vi "Main.vi"() -> ()   [LabVIEW 2020]
doc: "This is a home security Vi. Requires Arduino code for some some hardware that is implemented. It alerts the owner when someone enters the password wrong 5 times."
uses:
  Controls/Keyboard.ctl
  Controls/Door Animation.ctl
  Controls/Enum Control.ctl
  <vilib>/userdefined/High Color/IMAQdx.ctl
  <vilib>/MakerHub/LINX/Public/Peripherals/Digital/Digital Write N Chans.vi
  <vilib>/MakerHub/LINX/Private/Local IO/LinxDigitalWrite.vi
  <vilib>/MakerHub/LINX/Public/Utilities/Check Channel.vi
  <vilib>/MakerHub/LINX/Public/Utilities/Open Serial.vi
  <vilib>/MakerHub/LINX/Public/Sensors/Motion/Servo/Servo Open One Channel.vi
  <vilib>/MakerHub/LINX/Private/Utilties/Generate Error.vi
  <vilib>/MakerHub/LINX/Public/Sensors/Motion/Servo/Servo Close One Channel.vi
  <vilib>/MakerHub/LINX/LMH-LINX.lvlib
  <vilib>/vision/driver/NI_Vision_Acquisition_Software.lvlib
  <vilib>/MakerHub/LINX/Public/Sensors/Motion/Servo/Servo.lvlib
panel:
  out "RFID":bool
  in  "Arm/Disarm":bool
  in  "Door Animation":T1
  out "Denied":bool
  out "Granted":bool
  in  "Keyboard":T2
  out "Image":T3(plugin-control)
  in  "QR code":bool
  in  "stop":bool
  out "4x4 pound":string
  out "Passcode Entered":string
  in  "Serial Port":refnum<visa-resource-name>="COM3"
  # "Jaime Alvarez"
  # "ECE 144"
  # "1234 San Diego Bld"
  # "# 7"
  # "Scan your RFID, use QR code,\nor enter password manually\nto unlock the door. \nClap to Arm system or do it\nmanually."
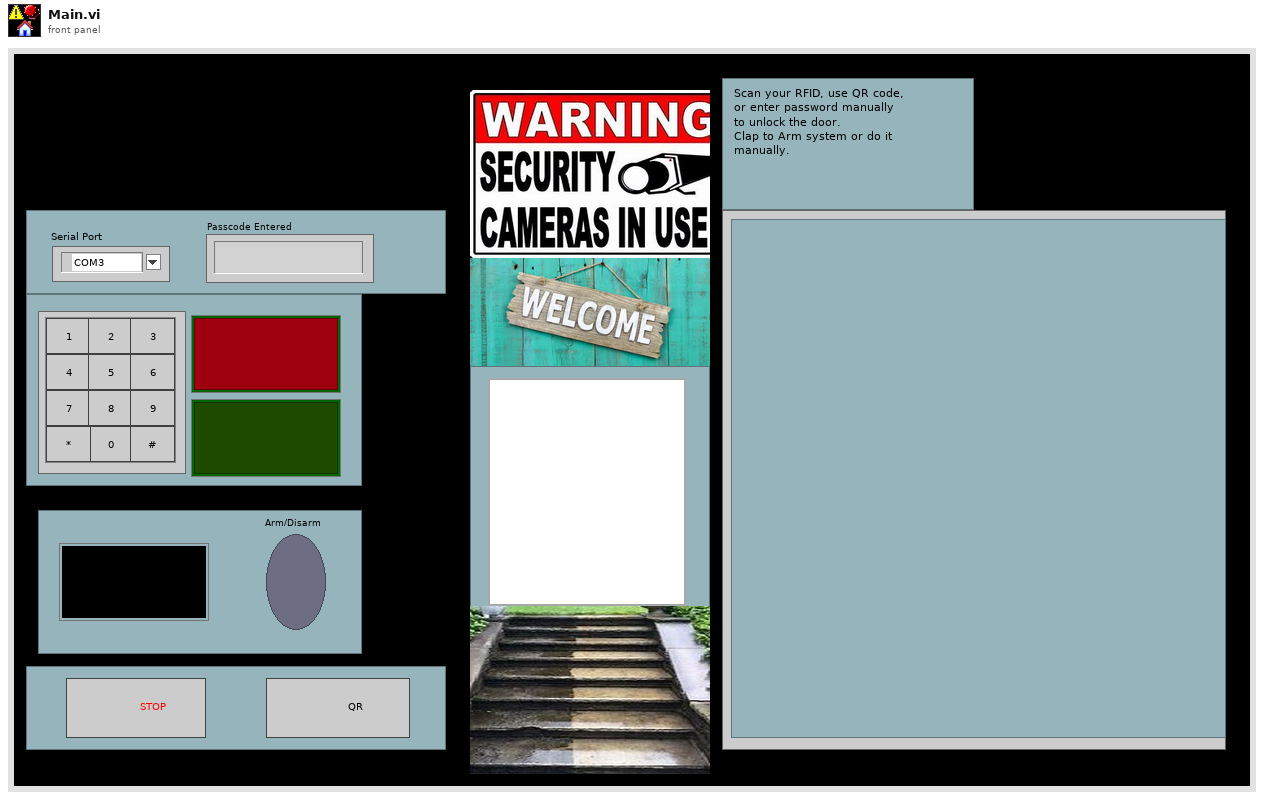
[diagram p1: front panel]
types:
  T1 = typedef "Door Animation.ctl" = u16
  T2 = typedef "Keyboard.ctl" = cluster{"Key 0":bool, "Key 1":bool, "Key 2":bool, "Key 3":bool, "Key 4":bool, "Key 5":bool, "Key 6":bool, "Key 7":bool, "Key 8":bool, "Key 9":bool, "Star Key":bool, "Pound Key":bool}
  T3 = typedef "IMAQ Image.ctl" = refnum<image>
  T4 = cluster{"Correct Song":i32[], "Wrong Song":i32[], "Wrong Beat":i32[]}
  T5 = cluster{"Key0":u8, "key1":u8, "Key2":u8, "Key3":u8, "Key4":u8, "Key5":u8, "Key6":u8, "Key7":u8, "Key8":u8, "Key9":u8, "Key*":u8, "Key#":u8, "Current Key":u8, "Total Code":u8}
  T6 = cluster{"Sound sensor":u8, "RGB":u8[], "Piezo Buzzer":i32, "Servo":i32}
  T7 = typedef "Enum Control.ctl" = enum16{"Initialize", "User Input", "Getting Keys", "Comparing Keys", "Correct Output", "Correct LED", "Wrong LED", "Wrong Output", "Too Many Tries", "Alert Owner", "Turn Off LED", "QR Code", "Stop"}
  T8 = typedef "LMH-LINX.lvlib/LINX Ref.ctl" = cluster{"IO":T9, "Interface":T10, "LINX Device Config":T11}
  T9 = typedef "LMH-LINX.lvlib/Platform.ctl" = enum16{"Remote", "Local"}
  T10 = typedef "LMH-LINX.lvlib/Interface.ctl" = enum16{"Serial", "TCP"}
  T11 = typedef "LMH-LINX.lvlib/Device.lvlib/LINX Device Config.ctl" = cluster{"Interface":T10, "COM Port":refnum<visa-resource-name>, "TCP Configuration":T12, "Device Family":u8, "Device ID":u8, "Device Name":string, "TCP Ref":refnum<k5>, "Channels":T13}
  T12 = typedef "LMH-LINX.lvlib/Device.lvlib/TCP Config.ctl" = cluster{"IP Address":string, "Port":u16}
  T13 = typedef "LMH-LINX.lvlib/Channels.ctl" = cluster{"DI":u8[], "DO":u8[], "AI":u8[], "AO":u8[], "PWM":u8[], "QE":u8[], "UART":u8[], "I2C 2":u8[], "SPI":u8[], "CAN":u8[], "Servo":u8[], "AI Ref (V)":dbl, "AI Resolution (Bits)":u8, "AO Ref (V)":dbl, "AO Resolution (Bits)":u8}
  T14 = enum8{"Enabled", "Disabled", "Disabled and Grayed Out"}
  T15 = typedef "IMAQdx.ctl" = refnum<k21>
  T16 = enum16{"T-Mobile", "AT&T", "Verizon", "Sprint", "Google-Fi"}
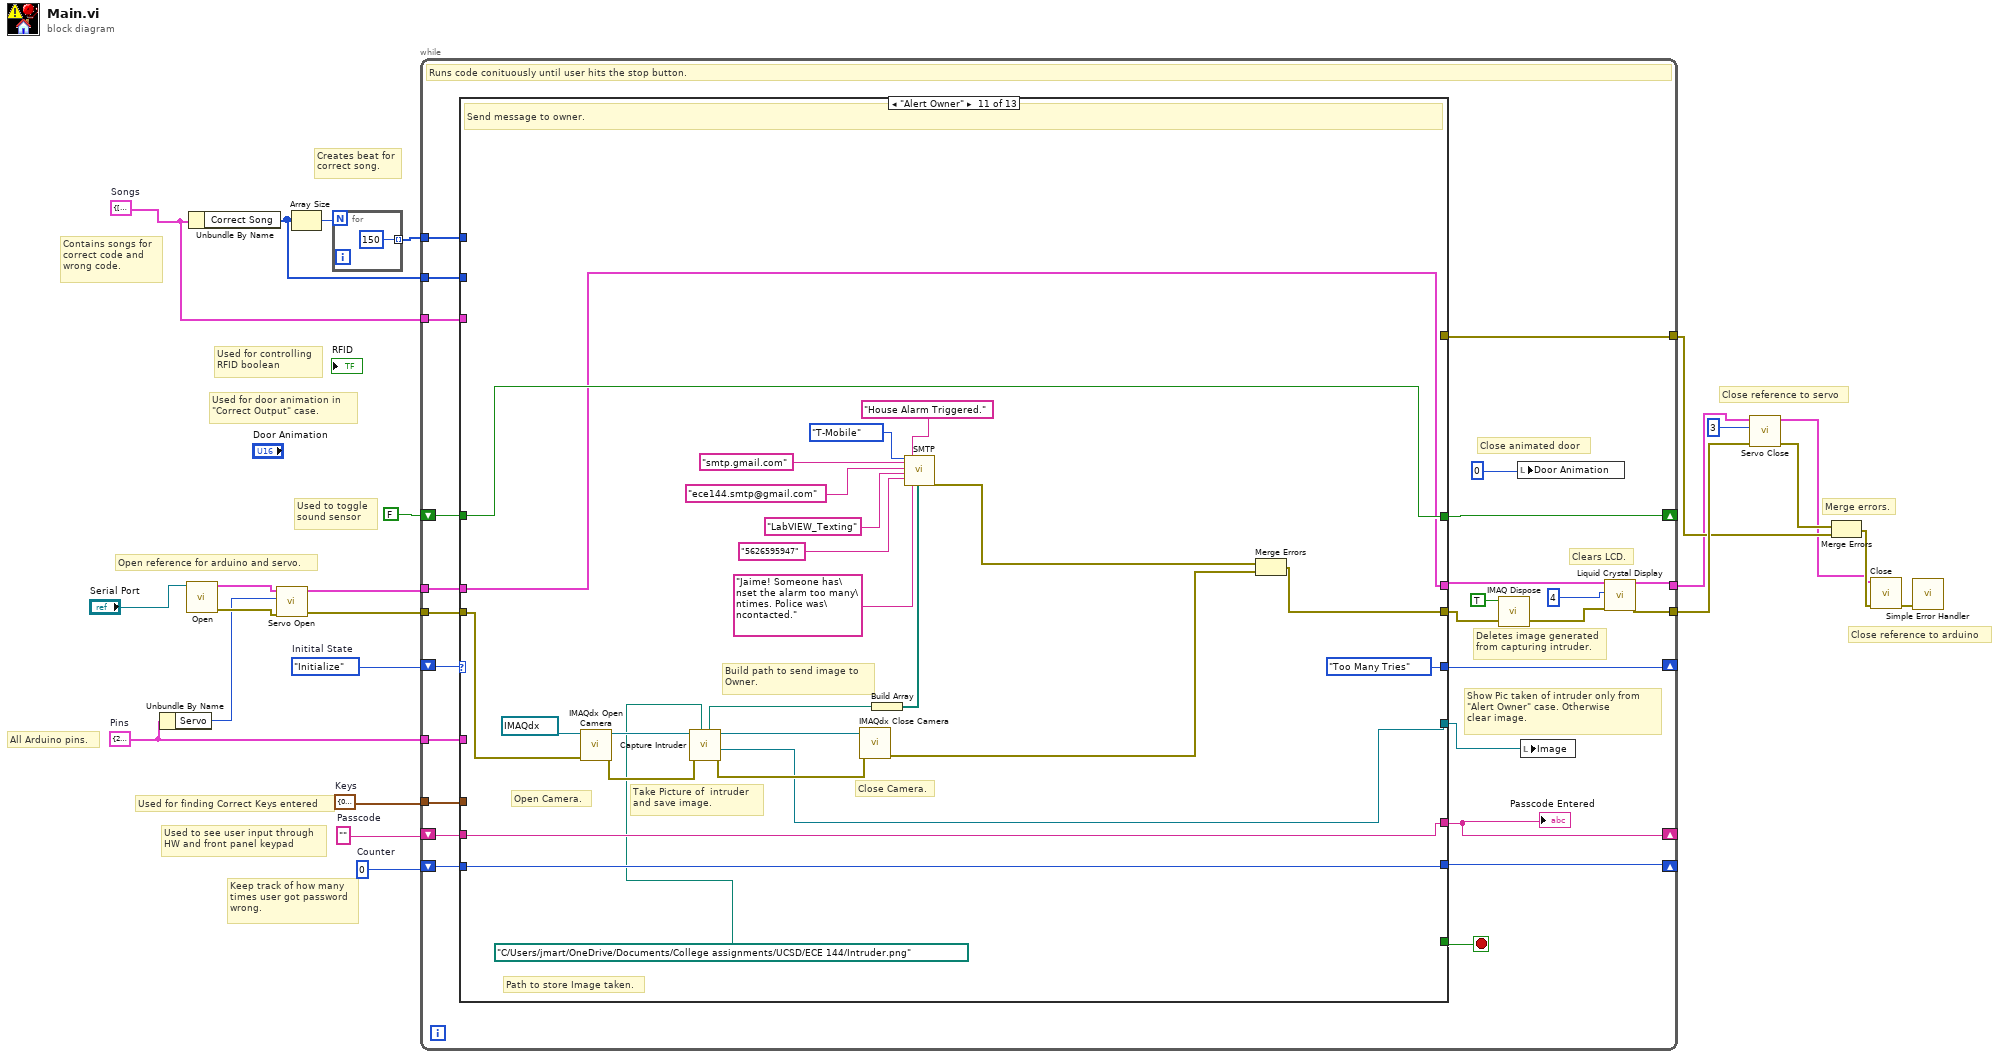
[diagram p0: block diagram]
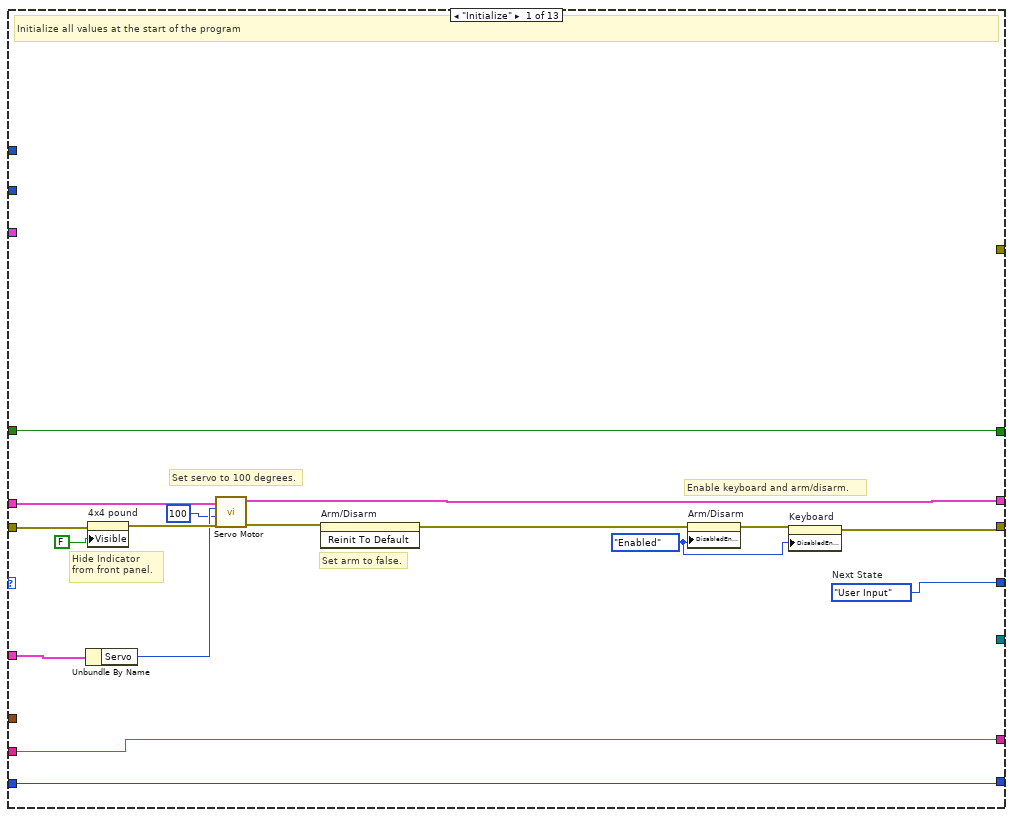
[diagram p2: hidden frame]
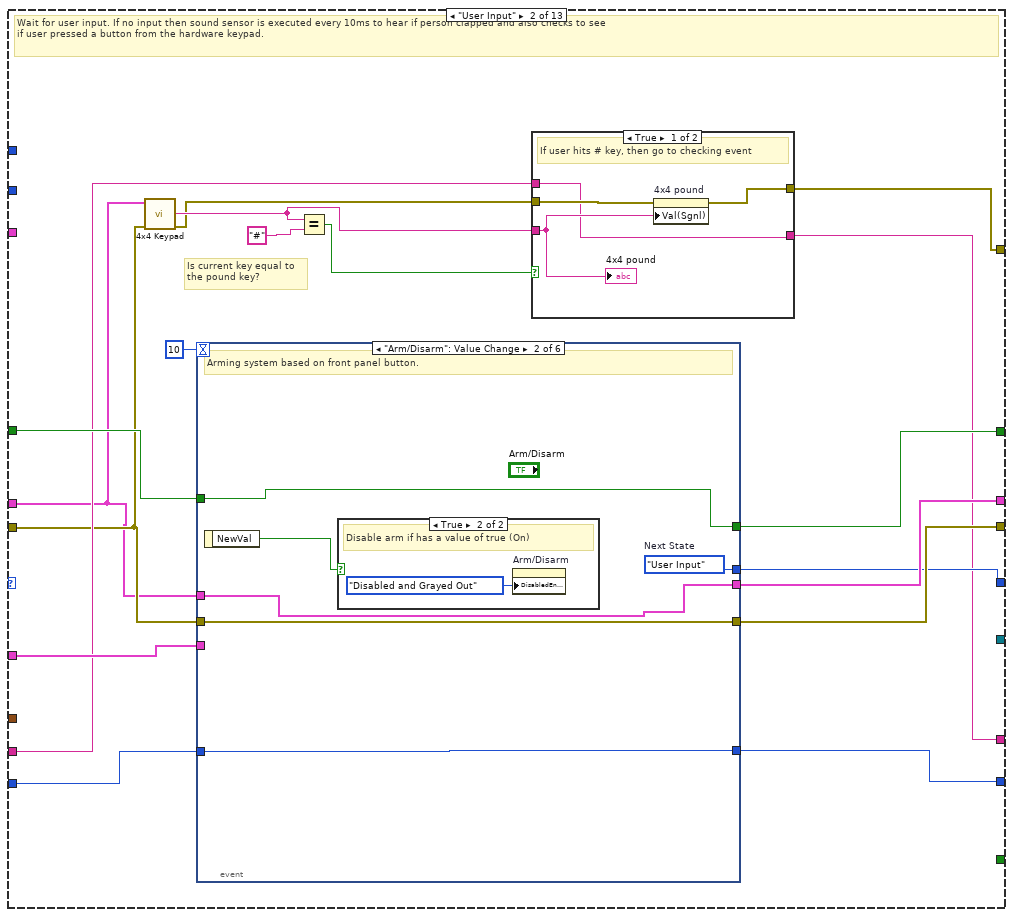
[diagram p3: hidden frame]
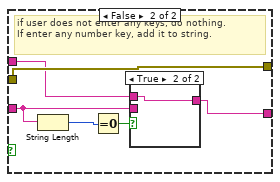
[diagram p4: hidden frame]
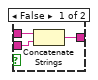
[diagram p5: hidden frame]
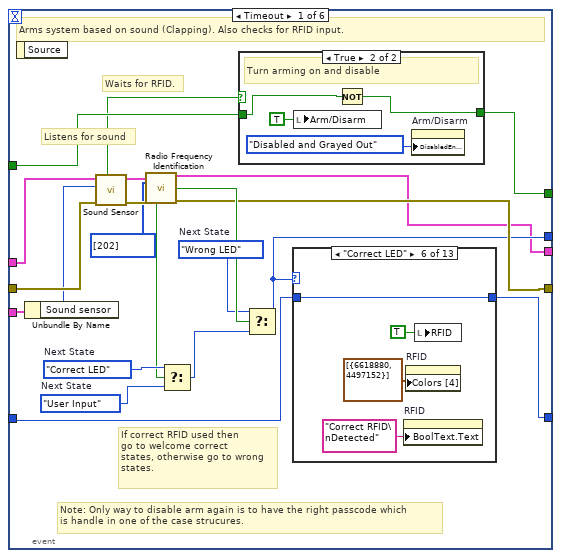
[diagram p6: hidden frame]
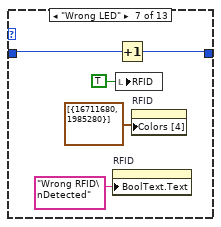
[diagram p12: hidden frame]
diagram:
  w13 = T4 {"Correct Song"=[1319, 1319, 0, 1319, 0, 1047, 1319, 0, 1568, 0, 0, 0, 784, 0, 0, 1568, 0, 0, 659, 0, 0, 880, 0, 988, 0, 932, 0, 880, 784, 1319, 1568, 1760, 0, 1397, 1568, 0, 1319, 0, 1568, 1175, 988, 0, 0], "Wrong Song"=[262, 523, 220, 440, 233, 466, 0, 0, 262, 523, 220, 440, 233, 466, 0, 0, 175, 349, 147, 294, 156, 311, 0, 0, 311, 277, 294, 277, 311, 311, 208, 208, 277, 262, 370, 349, 165, 466, 440, 415, 311, 247, 233, 220, 208, 0, 0, 0], "Wrong Beat"=[250, 250, 250, 250, 250, 250, 500, 1000, 250, 250, 250, 250, 250, 250, 500, 1000, 250, 250, 250, 250, 250, 250, 500, 1000, 250, 250, 250, 250, 250, 250, 500, 500, 250, 250, 250, 500, 500, 500, 500, 250, 250, 250, 250, 250, 250, 500, 500, 500]}  # Songs
  w19 = 0  # Counter
  w20 = ""  # Passcode
  w21 = T5 {"Key0"=0, "key1"=1, "Key2"=2, "Key3"=3, "Key4"=4, "Key5"=5, "Key6"=6, "Key7"=7, "Key8"=8, "Key9"=9, "Key*"=10, "Key#"=11, "Current Key"=0, "Total Code"=0}  # Keys
  w8 = T6 {"Sound sensor"=2, "RGB"=[45, 46, 47], "Piezo Buzzer"=9, "Servo"=3}  # Pins
  w23 = Enum_Control."Initialize"  # Initital State
  # "Used for controlling\nRFID boolean"
  # "Merge errors."
  # "Close reference to servo"
  # "Close reference to arduino"
  # "Contains songs for\ncorrect code and\nwrong code."
  # "Used for door animation in \n\"Correct Output\" case."
  # "Open reference for arduino and servo."
  # "Creates beat for\ncorrect song."
  # "Used to toggle \nsound sensor"
  # "Used to see user input through\nHW and front panel keypad"
  # "All Arduino pins."
  # "Used for finding Correct Keys entered"
  # "Keep track of how many\ntimes user got password\nwrong."
  n1 = Unbundle By Name(w8) -> ("Servo"=w7:i32)
  n2 = call-poly <vilib>:"Open.vi"("Serial Port"="Serial Port") -> ("Error Out"=w9:errorcluster, "LINX Resource"=w10:T8)  [unwired: 8 in, 1 out]
  n3 = Unbundle By Name(w13) -> ("Correct Song"=w14:i32[])
  n4 = call-poly <vilib>:"Servo Open.vi"("Error In"=w9, "Servo Channel"=w7, "LINX Resource"=w10) -> ("Error Out"=w11:errorcluster, "LINX Resource"=w12:T8)  [unwired: 7 in]
  n5 = Array Size(array=w14) -> (size(s)=w16:i32)
  n6 = for {
    N: w16 -> [_]
    tunnel: [150] -> w15 mode=indexing
  }
  n7 = while {
    shift-right: [w50] -> _
    shift-left: w23 -> [w51]
    tunnel: w12 -> [w49]
    tunnel: w11 -> [w48]
    shift-right: [w46] -> _
    shift-left: FALSE -> [w47]
    tunnel: [w39] -> w5
    tunnel: [w37] -> w2
    tunnel: w8 -> [w45]
    tunnel: w21 -> [w44]
    shift-right: [w42] -> _
    shift-left: w20 -> [w43]
    shift-right: [w40] -> _
    shift-left: w19 -> [w41]
    tunnel: [w35] -> w4
    tunnel: w15 -> [w33]
    tunnel: w14 -> [w32]
    tunnel: w13 -> [w31]
    stop <- w34 stop-if-true
    # "Deletes image generated\nfrom capturing intruder."
    # "Close animated door"
    # "Show Pic taken of intruder only from\n\"Alert Owner\" case. Otherwise\nclear image."
    # "Clears LCD."
    # "Runs code conituously until user hits the stop button."
    n8 = case shown="\"Alert Owner\"" w51 {
      tunnel: [w68 w82 w184 w200 w236 w252 w261 w304 w361 w403 Enum_Control."Too Many Tries" ("Initital State") Enum_Control."User Input" ("Initital State") w481] -> w50
      tunnel: w49 -> [w58 w70 w191 w199 w247 w257 w275 w299 w359 w401 w441 w476 w483]
      tunnel: w48 -> [w60 w71 w190 w215 w245 _ w272 w298 w356 w373 w436 w474 w482]
      tunnel: w47 -> [w67 w85 w192 w206 w248 w251 w268 w292 w362 w374 w454 w471 w484]
      tunnel: [w67 w80 w192 w206 w248 w251 w268 w292 w362 w374 w454 w471 w484] -> w46
      tunnel: [w61 w83 w185 w214 w244 w249 w266 w279 w344 w366 w444 w462 w482] -> w27
      tunnel: [w57 w84 w191 w199 w247 w253 w270 w276 w343 w387 w441 w475 w483] -> w36
      tunnel: [_ _ _ _ _ _ _ _ _ _ _ _ TRUE] -> w34
      tunnel: w45 -> [w54 w81 _ _ _ w256 w274 w284 _ w380 _ w478 _]
      tunnel: w44 -> [_ _ w189 _ _ _ _ _ _ _ _ _ _]
      tunnel: w43 -> [w65 w73 w188 w207 w235 w255 w269 w303 w360 w402 w452 w466 _]
      tunnel: [w65 w72 w178 w207 w243 w255 w269 w303 w360 w402 w452 w466 "" ("Passcode")] -> w42
      tunnel: w41 -> [w64 w79 w183 w208 w240 w254 w260 _ w341 _ w451 w470 _]
      tunnel: [w64 w78 w183 w208 w240 w254 w260 0 ("Counter") w341 0 ("Counter") w451 w470 0 ("Counter")] -> w40
      tunnel: [_ w69 _ _ _ _ _ w280 _ w375 _ _ _] -> w35
      tunnel: w33 -> [_ _ _ _ _ _ _ w291 _ _ _ _ _]
      tunnel: w32 -> [_ _ _ _ _ _ _ w290 _ _ _ _ _]
      tunnel: w31 -> [_ _ _ _ _ _ _ _ _ w381 _ _ _]
      tunnel: [_ _ _ _ _ _ _ _ _ _ w442 _ _] -> w29
      frame "Initialize" {
        w62 = T14."Enabled" ("Disabled")
        w68 = Enum_Control."User Input"  # Next State
        # "Set servo to 100 degrees."
        # "Set arm to false."
        # "Enable keyboard and arm/disarm."
        # "Hide Indicator\nfrom front panel."
        # "Initialize all values at the start of the program"
        n9 = Unbundle By Name(w54) -> ("Servo"=w53:i32)
        n10 = property on="4x4 pound" class="Str"(error in=w60, "Visible"=FALSE) -> (error out=w56:errorcluster)  [unwired: 1 in, 1 out]
        n11 = call "Servo Motor.vi"("Error In"=w56, "Position"=100, "Servo Channel"=w53, "LINX Resource In"=w58) -> ("Error Out"=w55:errorcluster, "LINX Resource Out"=w57:T8)  [unwired: 5 in, 1 out]
        n12 = invoke on="Arm/Disarm" class="Bool (strict)" method="Reinit To Default"(error in=w55) -> (error out=w66:errorcluster)  [unwired: 2 in, 2 out]
        n13 = property on="Arm/Disarm" class="Bool (strict)"(error in=w66, "DisabledEnum"=w62) -> (error out=w63:errorcluster)  [unwired: 1 in, 1 out]
        n14 = property on="Keyboard" class="Clust (strict)"(error in=w63, "DisabledEnum"=w62) -> (error out=w61:errorcluster)  [unwired: 1 in, 1 out]
      }
      frame "User Input" {
        # "Is current key equal to \nthe pound key?"
        # "Wait for user input. If no input then sound sensor is executed every 10ms to hear if person clapped and also checks to see\nif user pressed a button from the hardware keypad."
        n15 = call "4x4 Keypad.vi"("Error In"=w71, "LINX Resource"=w70) -> ("Error Out"=w74:errorcluster, "string out"=w75:string)  [unwired: 7 in, 1 out]
        n16 = event shown="[1] \"Arm/Disarm\": Value Change" {
          selector: _ -> [_ _ _ _ _ _]
          dyn-events: _ -> [_ _ _ _ _ _]
          timeout: 10 -> [_ _ _ _ _ _]
          tunnel: [w104 w152 w159 w166 w169 w177] -> w82
          tunnel: w85 -> [w119 w147 w154 w162 w172 w176]
          tunnel: w70 -> [w121 w148 w156 w161 w171 w175]
          tunnel: w71 -> [w120 w149 w155 w160 w170 w174]
          tunnel: [w118 w147 w154 w162 w172 w176] -> w80
          tunnel: [w101 w148 w156 w161 w171 w175] -> w84
          tunnel: [w106 w149 w155 w160 w170 w174] -> w83
          tunnel: w81 -> [w117 _ _ _ _ _]
          tunnel: w79 -> [w105 w150 w157 w164 w168 w173]
          tunnel: [w103 w150 w157 w163 w167 w173] -> w78
          event Timeout {
            w108 = Enum_Control."Wrong LED"  # Next State
            w112 = Enum_Control."Correct LED"  # Next State
            w111 = Enum_Control."User Input"  # Next State
            # "Waits for RFID."
            # "Listens for sound"
            # "If correct RFID used then \ngo to welcome correct\nstates, otherwise go to wrong\nstates."
            # "Note: Only way to disable arm again is to have the right passcode which\nis handle in one of the case strucures."
            # "Arms system based on sound (Clapping). Also checks for RFID input."
            n17 = event-data() -> ()  [unwired: 1 in, 1 out]
            n18 = Unbundle By Name(w117) -> ("Sound sensor"=w116:u8)
            n19 = call "Sound Sensor.vi"("Error In"=w120, "DI Channel"=w116, "LINX Resource In"=w121) -> ("Error Out"=w114:errorcluster, "Sound?"=w113:bool, "LINX Resource Out"=w115:T8)  [unwired: 6 in]
            n20 = call "Radio Frequency Identification.vi"("LINX Resource"=w115, "RFID Value"=u8[] [202], "Error In"=w114) -> ("LINX Resource Out"=w101:T8, "Wrong ID"=w109:bool, "Correct ID"=w107:bool, "Error Out"=w106:errorcluster)  [unwired: 8 in, 1 out]
            n21 = Select(t=w112, s=w107, f=w111) -> (s? t:f=w110:T7)
            n22 = case shown="True" w113 {
              tunnel: w119 -> [w142 w145]
              tunnel: [w142 w146] -> w118
              frame False {
                # "Do nothing."
              }
              frame True {
                # "Turn arming on and disable"
                n23 = local write "Arm/Disarm"(TRUE ("Arm/Disarm")) -> ()
                n24 = Not(x=w145) -> (.not. x?=w146:bool)
                n25 = property on="Arm/Disarm" class="Bool (strict)"("DisabledEnum"=T14."Disabled and Grayed Out" ("Disabled")) -> ()  [unwired: 2 in, 2 out]
              }
            }
            n26 = Select(t=w108, s=w109, f=w110) -> (s? t:f=w104:T7)
            n27 = case shown="\"Correct LED\"" w104 {
              tunnel: w105 -> [w122 w123 w124 w125 w126 w130 w135 w136 w137 w138 w139 w140 w141]
              tunnel: [w122 w123 w124 w125 w126 w130 w134 w136 w137 w138 w139 w140 w141] -> w103
              frame "Initialize" {
              }
              frame "User Input" {
              }
              frame "Getting Keys" {
              }
              frame "Comparing Keys" {
              }
              frame "Correct Output" {
              }
              frame "Correct LED" {
                n28 = property on="RFID" class="Bool (strict)"("BoolText.Text"="Correct RFID\nDetected" ("Boolean Text.Text")) -> ()  [unwired: 2 in, 2 out]
                n29 = property on="RFID" class="Bool (strict)"("Colors [4]"=cluster{u32, u32}[] [{6618880, 4497152}]) -> ()  [unwired: 2 in, 2 out]
                n30 = local write "RFID"(TRUE ("RFID")) -> ()
              }
              frame "Wrong LED" {
                n31 = property on="RFID" class="Bool (strict)"("BoolText.Text"="Wrong RFID\nDetected" ("Boolean Text.Text")) -> ()  [unwired: 2 in, 2 out]
                n32 = local write "RFID"(TRUE ("RFID")) -> ()
                n33 = Increment(x=w135) -> (x+1=w134:i32)
                n34 = property on="RFID" class="Bool (strict)"("Colors [4]"=cluster{u32, u32}[] [{16711680, 1985280}]) -> ()  [unwired: 2 in, 2 out]
              }
              frame "Wrong Output" {
              }
              frame "Too Many Tries" {
              }
              frame "QR Code" {
              }
              frame "Stop" {
              }
              frame "Turn Off LED" {
              }
              frame "Alert Owner" {
              }
            }
          }
          event "Arm/Disarm": Value Change {
            w152 = Enum_Control."User Input"  # Next State
            # "Arming system based on front panel button."
            n35 = event-data() -> ("NewVal"=w151:bool)  [unwired: 1 in]
            n36 = case shown="True" w151 {
              frame False {
                # "Do nothing"
              }
              frame True {
                # "Disable arm if has a value of true (On)"
                n37 = property on="Arm/Disarm" class="Bool (strict)"("DisabledEnum"=T14."Disabled and Grayed Out" ("Disabled")) -> ()  [unwired: 2 in, 2 out]
              }
            }
          }
          event Value Change {
            w159 = Enum_Control."Getting Keys"  # Next State
            # "This gives time for buttons on the front\npanel to change color to show that it is being pressed."
            # "User presses a button on the front panel keyboard"
            n38 = event-data() -> ()  [unwired: 1 in, 1 out]
            n39 = Wait (ms)(milliseconds to wait=u32 20) -> ()  [unwired: 1 out]
          }
          event "4x4 pound": Value Change {
            w166 = Enum_Control."Comparing Keys"  # Initital State
            # "Use counter to keep track of how many times user\nentered the wrong passcode."
            # "User pressed pound key to submit their passcode for entry/denial."
            n40 = event-data() -> ()  [unwired: 1 in, 1 out]
            n41 = Wait (ms)(milliseconds to wait=u32 20) -> ()  [unwired: 1 out]
            n42 = Increment(x=w164) -> (x+1=w163:i32)
          }
          event "QR code": Value Change {
            w169 = Enum_Control."QR Code"  # Next State
            # "User wants to use QR code to try to enter home."
            n43 = event-data() -> ()  [unwired: 1 in, 1 out]
            n44 = Increment(x=w168) -> (x+1=w167:i32)
          }
          event "stop": Value Change {
            w177 = Enum_Control."Stop"  # Initital State
            # "Stop system."
            n45 = event-data() -> ()  [unwired: 1 in, 1 out]
          }
        }
        n46 = Equal?(x=w75, y="#") -> (x = y?=w76:bool)
        n47 = case shown="True" w76 {
          tunnel: [w88 w93] -> w69
          tunnel: w75 -> [w89 w94]
          tunnel: w74 -> [w90 w93]
          tunnel: [w87 w91] -> w72
          tunnel: w73 -> [w87 w92]
          frame True {
            # "If user hits # key, then go to checking event"
            n48 = property on="4x4 pound" class="Str"(error in=w90, "Val(Sgnl)"=w89) -> (error out=w88:errorcluster)  [unwired: 1 in, 1 out]
            "4x4 pound" <- w89
          }
          frame False {
            # "if user does not enter any keys, do nothing.\nIf enter any number key, add it to string."
            n49 = String Length(string=w94) -> (length=w96:i32)
            n50 = Equal To 0?(x=w96) -> (x = 0?=w95:bool)
            n51 = case shown="True" w95 {
              tunnel: w94 -> [w99 _]
              tunnel: [w98 w100] -> w91
              tunnel: w92 -> [w97 w100]
              frame False {
                n52 = Concatenate Strings(w97, w99) -> (w98:string)
              }
              frame True {
              }
            }
          }
        }
      }
      frame "Getting Keys" {
        w184 = Enum_Control."User Input"  # Initital State
        # "Set button back to false.\nCreate dependents."
        # "Concatenate Strings."
        # "Find button pressed and \nconvert number to string."
        # "Convert cluster to array\nand search index of button pressed."
        # "Get the users input keys and display them as a string back to the user."
        n53 = Cluster To Array(cluster=w189) -> (array=w182:u8[])
        n54 = property on="Keyboard" class="Clust (strict)"(error in=w190) -> (error out=w186:errorcluster, "Value"=w195:T2)  [unwired: 1 in, 1 out]
        n55 = Cluster To Array(cluster=w195) -> (array=w193:bool[])
        n56 = Search 1D Array(1D array=w193, element=TRUE) -> (index of element=w180:i32)  [unwired: 1 in]
        n57 = Index Array(array=w182, index=w180) -> (element=w179:u8)
        n58 = Number To Decimal String(number=w179) -> (decimal integer string=w181:string)  [unwired: 1 in]
        n59 = Concatenate Strings(w188, w181) -> (w187:string)
        n60 = flat-sequence {
          tunnel: w187 -> [w198]
          tunnel: [w198] -> w178
          tunnel: w186 -> [w197]
          tunnel: [w196] -> w185
          frame #0 {
            n61 = invoke on="Keyboard" class="Clust (strict)" method="Reinit To Default"(error in=w197) -> (error out=w196:errorcluster)  [unwired: 2 in, 2 out]
          }
        }
      }
      frame "QR Code" {
        w201 = Enum_Control."Wrong LED"  # Next State
        w202 = Enum_Control."Correct LED"  # Next State
        # "If data of QR Code matches string, then go to correct LED, otherwise it's the wrong QR Code."
        # "Run until QR code \nis found."
        # "Close Camera and dispose\nimage."
        # "Create Location\nto store image."
        # "Open Camera and grab \nacquisition"
        # "Finds QR code and determines if it's valid."
        n62 = call <vilib>:"IMAQdx Open Camera.vi"("error in"=w215, "Session In"=T15 "cam0") -> ("error out"=w222:errorcluster, "Session Out"=w221:T15)  [unwired: 8 in]
        n63 = call <vilib>:"IMAQdx Configure Grab.vi"("error in"=w222, "Session In"=w221) -> ("error out"=w219:errorcluster, "Session Out"=w211:T15)  [unwired: 8 in]
        n64 = call "IMAQ Create"("Image Name"="Current Image", "error in (no error)"=w219) -> ("New Image"=w210:T3, "error out"=w209:errorcluster)  [unwired: 3 in]
        n65 = while {
          tunnel: [w230] -> w213
          tunnel: [w224] -> w212
          tunnel: w211 -> [w229]
          tunnel: w210 -> [w228]
          tunnel: w209 -> [w227]
          tunnel: [w225] -> w205
          stop <- w226 stop-if-true
          n66 = call "QR  Code.vi"("Session In"=w229, "Image In"=w228, "error in"=w227) -> ("Session Out"=w224:T15, "Found?"=w226:bool, "Image"=→"Image":T3, "Data"=w225:string, "error out"=w230:errorcluster)  [unwired: 8 in]
        }
        n67 = Equal?(x=w205, y="Access Granted! Welcome home, Jaime.") -> (x = y?=w203:bool)
        n68 = Select(t=w202, s=w203, f=w201) -> (s? t:f=w200:T7)
        n69 = call <vilib>:"IMAQdx Close Camera.vi"("error in"=w213, "Session In"=w212) -> ("error out"=w217:errorcluster)  [unwired: 9 in]
        n70 = call "IMAQ Dispose"("All Images? (No)"=TRUE, "error in (no error)"=w217) -> ("error out"=w214:errorcluster)  [unwired: 4 in]
      }
      frame "Comparing Keys" {
        w237 = Enum_Control."Alert Owner"  # Next State
        w241 = Enum_Control."Correct LED"  # Next State
        w242 = Enum_Control."Wrong LED"  # Next State
        w246 = "12345"  # Correct Passcode
        # "Delete values from indicator displayed\nto the user."
        # "If users used all their tries,\nthen go to 'Alert Owner'\nstate."
        # "If entered correct code, go to correct LED."
        # "If user enters 5 times wrong \nthen send alarm."
        # "Turn pound key back to false"
        # "Compares to see if the users keys entered is the right passcode."
        n71 = invoke on="Keyboard" class="Clust (strict)" method="Reinit To Default"(error in=w245) -> (error out=w244:errorcluster)  [unwired: 2 in, 2 out]
        n72 = String Length(string=w235) -> (length=w231:i32)
        n73 = Equal?(x=w246, y=w235) -> (x = y?=w233:bool)
        n74 = Replace Substring(2:w231, 4:"" ("substring (\"\")"), 5:w235) -> (1:w243:string)  [unwired: 1 in, 1 out]
        n75 = Select(t=w241, s=w233, f=w242) -> (s? t:f=w238:T7)
        n76 = Equal?(x=5 ("length (len. of substring)"), y=w240) -> (x = y?=w239:bool)
        n77 = Select(t=w237, s=w239, f=w238) -> (s? t:f=w236:T7)
      }
      frame "Correct LED" {
        w252 = Enum_Control."Correct Output"  # Next State
        # "Turn on front Panel LED."
        # "Turn on Red LED."
        # "Red = Off\nGreen = On\nBlue = Off"
        # "Light up green LED from RGB."
        n78 = Unbundle By Name(w256) -> ("RGB"=w258:u8[])
        n79 = call-poly <vilib>:"Digital Write.vi"("Values"=bool[] [FALSE, TRUE, FALSE], "DO Channels"=w258, "LINX Resource"=w257) -> ("Error Out"=w249:errorcluster, "LINX Resource"=w253:T8)  [unwired: 7 in]
        "Granted" <- TRUE ("Granted")
      }
      frame "Wrong LED" {
        w262 = Enum_Control."Alert Owner"  # Next State
        w263 = Enum_Control."Wrong Output"  # Next State
        # "If tried 5 times, then too many times already\nNote: This is alread handled in another case, but this\none ensures that it works for the QR and RFID"
        # "Turn on front panel LED."
        # "Turn on Red LED."
        # "Red = On\nGreen = Off\nBlue = Off"
        # "Turn on Red LED from RGB."
        n80 = Unbundle By Name(w274) -> ("RGB"=w273:u8[])
        n81 = call-poly <vilib>:"Digital Write.vi"("Error In"=w272, "Values"=bool[] [TRUE, FALSE, FALSE], "DO Channels"=w273, "LINX Resource"=w275) -> ("Error Out"=w266:errorcluster, "LINX Resource"=w270:T8)  [unwired: 6 in]
        n82 = Equal?(x=5, y=w260) -> (x = y?=w264:bool)
        n83 = Select(t=w262, s=w264, f=w263) -> (s? t:f=w261:T7)
        "Denied" <- TRUE ("Denied")
      }
      frame "Correct Output" {
        w282 = 101
        w305 = Enum_Control."Turn Off LED"  # Next State
        # "These two loops operates the physical door controlled by the servo motor."
        # "Piezo Buzzer: Play song when user gets correct password."
        # "Reset\nCounter."
        # "LCD: Send greetings to LCD"
        # "Waits for user to press okay on dialog box."
        # "Enable the Arm when entered right passcode."
        # "Display welcome signs through LCD and dialog box. Also play song on Piezo Buzzer and moves servo."
        n84 = Unbundle By Name(w284) -> ("Piezo Buzzer"=w289:i32)
        n85 = Unbundle By Name(w284) -> ("Servo"=w278:i32)
        n86 = property on="Arm/Disarm" class="Bool (strict)"("DisabledEnum"=T14."Enabled" ("Disabled")) -> ()  [unwired: 2 in, 2 out]
        n87 = call "Liquid Crystal Display.vi"("LINX Resource In"=w299, "string"="Welcome ", "string 2"="Home, Jaime.", "Error In"=w298) -> ("LINX Resource Out"=w286:T8, "string"=w295:string, "string 2"=w294:string, "Error Out"=w285:errorcluster)  [unwired: 11 in, 1 out]
        n88 = Concatenate Strings(w295, w294) -> (w293:string)
        n89 = for {
          N: w282 -> [_]
          tunnel: w286 -> [w322]
          tunnel: w285 -> [w321]
          tunnel: w278 -> [w314]
          tunnel: [w317] -> w283
          tunnel: [w316] -> w281
          tunnel: [w314] -> w277
          i -> [w319]
          # "Open Door"
          n90 = Subtract(x=100, y=w319) -> (x-y=w318:i32)
          n91 = call "Servo Motor.vi"("Error In"=w321, "Position"=w318, "Servo Channel"=w314, "LINX Resource In"=w322) -> ("Error Out"=w316:errorcluster, "LINX Resource Out"=w317:T8)  [unwired: 5 in, 1 out]
          n92 = Wait (ms)(milliseconds to wait=u32 25) -> ()  [unwired: 1 out]
        }
        n93 = for {
          N: 5 -> [_]
          shift-right: [w324] -> _
          shift-left: u16 0 -> [w325]
          # "Open animated door."
          n94 = local write "Door Animation"(w325) -> ()
          n95 = Increment(x=w325) -> (x+1=w324:u16)
          n96 = Wait (ms)(milliseconds to wait=u32 100) -> ()  [unwired: 1 out]
        }
        n97 = for {
          tunnel: w291 -> [w329] mode=indexing
          tunnel: w290 -> [w328] mode=indexing
          tunnel: w289 -> [w331]
          tunnel: [w330] -> w280
          tunnel: w286 -> [w327]
          tunnel: w285 -> [w326]
          # "Play song."
          n98 = Equal To 0?(x=w328) -> (x = 0?=w332:bool)
          n99 = case shown="False" w332 {
            tunnel: w329 -> [w334 w338]
            tunnel: w331 -> [_ w340]
            tunnel: w328 -> [_ w339]
            tunnel: [w333 w337] -> w330
            tunnel: w327 -> [_ w336]
            tunnel: w326 -> [w333 w335]
            frame True {
              # "Pause."
              n100 = Wait (ms)(milliseconds to wait=w334) -> ()  [unwired: 1 out]
            }
            frame False {
              # "Play Chord with relative beat."
              n101 = call "Piezo Buzzer.vi"("Duration (ms)"=w338, "Error In"=w335, "Frequency (Hz)"=w339, "Channel"=w340, "LINX Resource"=w336) -> ("Error Out"=w337:errorcluster)  [unwired: 5 in, 1 out]
              n102 = Wait (ms)(milliseconds to wait=w338) -> ()  [unwired: 1 out]
            }
          }
        }
        n103 = for {
          N: w282 -> [_]
          tunnel: w283 -> [w313]
          tunnel: w281 -> [w311]
          tunnel: [w310] -> w279
          tunnel: [w308] -> w276
          tunnel: w277 -> [w307]
          i -> [w312]
          # "Close Door"
          n104 = call "Servo Motor.vi"("Error In"=w311, "Position"=w312, "Servo Channel"=w307, "LINX Resource In"=w313) -> ("Error Out"=w310:errorcluster, "LINX Resource Out"=w308:T8)  [unwired: 5 in, 1 out]
          n105 = Wait (ms)(milliseconds to wait=u32 25) -> ()  [unwired: 1 out]
        }
        n106 = One Button Dialog(message=w293) -> (true=w306:bool)  [unwired: 1 in]
        n107 = Select(t=w305, s=w306, f=Enum_Control."Correct Output") -> (s? t:f=w304:T7)
      }
      frame "Wrong Output" {
        w347 = "\r\n"
        w363 = Enum_Control."Turn Off LED"  # Next State
        # "Count down on \ntries left."
        # "Formats LCD string to send to \ndialog box."
        # "Display warning to LCD."
        # "Waits for user to hit okay on \ndialog box."
        # "Sends warning to LCD and dialog box if user gets passcode wrong."
        n108 = Subtract(x=5, y=w341) -> (x-y=w346:i32)
        n109 = Build Array(w346) -> (w355:i32[])
        n110 = call "Liquid Crystal Display.vi"("LINX Resource In"=w359, "string"="Wrong Code.", "Data"=w355, "string 2"=" Tries Left.", "Error In"=w356) -> ("LINX Resource Out"=w343:T8, "string"=w352:string, "Response"=w354:u8[], "string 2"=w351:string, "Error Out"=w345:errorcluster)  [unwired: 10 in]
        n111 = Index Array(array=w354, index=0) -> (element=w348:u8)
        n112 = Format Into String(format string="%s %d %s %s", initial string=w352, error in=w345, w347, w348, w351, w347) -> (resulting string=w350:string, error out=w344:errorcluster)
        n113 = One Button Dialog(message=w350) -> (true=w365:bool)  [unwired: 1 in]
        n114 = Select(t=w363, s=w365, f=Enum_Control."Wrong Output") -> (s? t:f=w361:T7)
      }
      frame "Too Many Tries" {
        w388 = T14."Enabled" ("Disabled")
        w391 = T14."Disabled and Grayed Out" ("Disabled")
        w404 = Enum_Control."User Input"  # Next State
        # "Arm the system even if it was not armed. This is because the owner might forgot to arm\n it and if someone triggers the alarm then we want the system to be secured."
        # "Text to Dialog box, then go to \nnext state."
        # "Enable all controls."
        # "Disable all controls so user cannot use it anymore.\nfor the amount of time it takes for song to play."
        # "Piezo Buzzer: Play song when user tries too many time (Alarm)."
        # "Reset \nCounter."
        # "Send Message to LCD"
        # "Displays intruder Alert, flashes front panel LED and RBG, plays alarm."
        n115 = Unbundle By Name(w381) -> ("Wrong Song"=w382:i32[])
        n116 = Unbundle By Name(w381) -> ("Wrong Beat"=w378:i32[])
        n117 = Unbundle By Name(w380) -> ("Piezo Buzzer"=w379:i32)
        n118 = call "Liquid Crystal Display.vi"("LINX Resource In"=w401, "string"="Intruder! ", "string 2"="Alerting Owner!", "Error In"=w373) -> ("LINX Resource Out"=w376:T8, "string"=w398:string, "string 2"=w397:string, "Error Out"=w395:errorcluster)  [unwired: 11 in, 1 out]
        n119 = Unbundle By Name(w380) -> ("RGB"=w386:u8[])
        n120 = Concatenate Strings(w398, w397) -> (w396:string)
        n121 = property on="Keyboard" class="Clust (strict)"(error in=w395, "DisabledEnum"=w391) -> (error out=w394:errorcluster)  [unwired: 1 in, 1 out]
        n122 = local write "Arm/Disarm"(TRUE ("Arm/Disarm")) -> ()
        n123 = property on="stop" class="Bool"(error in=w394, "DisabledEnum"=w391) -> (error out=w393:errorcluster)  [unwired: 1 in, 1 out]
        n124 = property on="Arm/Disarm" class="Bool (strict)"(error in=w393, "DisabledEnum"=w391) -> (error out=w392:errorcluster)  [unwired: 1 in, 1 out]
        n125 = property on="QR code" class="Bool"(error in=w392, "DisabledEnum"=w391) -> (error out=w377:errorcluster)  [unwired: 1 in, 1 out]
        n126 = for {
          N: 160 -> [_]
          tunnel: w376 -> [w435]
          tunnel: [w434] -> w387
          tunnel: w386 -> [w433]
          shift-right: [w432] -> _
          shift-left: bool[] [TRUE, FALSE, FALSE] ("Values") -> [w429]
          tunnel: [w426] -> w372
          tunnel: w377 -> [w430]
          # "Flash red LED"
          n127 = Index Array(array=w429, index=0) -> (element=w425:bool)
          n128 = call "Flashing Warning RGB.vi"("error in (no error)"=w430, "Values"=w429, "RGB"=w433, "LINX Resource Out"=w435) -> ("error out"=w427:errorcluster, "Array"=w432:bool[], "LINX Resource"=w434:T8)  [unwired: 5 in]
          n129 = property on="Denied" class="Bool (strict)"(error in=w427, "Value"=w425) -> (error out=w426:errorcluster)  [unwired: 1 in, 1 out]
          n130 = Wait (ms)(milliseconds to wait=u32 100) -> ()  [unwired: 1 out]
        }
        n131 = for {
          tunnel: [w413] -> _
          tunnel: [w412] -> w375
          tunnel: w382 -> [w410] mode=indexing
          tunnel: w379 -> [w411]
          tunnel: w378 -> [w409] mode=indexing
          tunnel: w377 -> [w408]
          tunnel: w376 -> [w407]
          # "Play song"
          n132 = Equal To 0?(x=w410) -> (x = 0?=w414:bool)
          n133 = case shown="False" w414 {
            tunnel: [w416 w424] -> w413
            tunnel: [w415 w423] -> w412
            tunnel: w411 -> [_ w422]
            tunnel: w410 -> [_ w421]
            tunnel: w409 -> [w417 w420]
            tunnel: w408 -> [w415 w419]
            tunnel: w407 -> [w416 w418]
            frame True {
              # "Pause for one beat."
              n134 = Wait (ms)(milliseconds to wait=w417) -> ()  [unwired: 1 out]
            }
            frame False {
              # "Play not for relative beat."
              n135 = call "Piezo Buzzer.vi"("Duration (ms)"=w420, "Error In"=w419, "Frequency (Hz)"=w421, "Channel"=w422, "LINX Resource"=w418) -> ("Error Out"=w423:errorcluster, "LINX Resource Out"=w424:T8)  [unwired: 5 in]
              n136 = Wait (ms)(milliseconds to wait=w420) -> ()  [unwired: 1 out]
            }
          }
        }
        n137 = One Button Dialog(message=w396) -> (true=w406:bool)  [unwired: 1 in]
        n138 = property on="QR code" class="Bool"(error in=w372, "DisabledEnum"=w388) -> (error out=w390:errorcluster)  [unwired: 1 in, 1 out]
        n139 = Select(t=w404, s=w406, f=Enum_Control."Too Many Tries") -> (s? t:f=w403:T7)
        n140 = property on="stop" class="Bool"(error in=w390, "DisabledEnum"=w388) -> (error out=w389:errorcluster)  [unwired: 1 in, 1 out]
        n141 = property on="Keyboard" class="Clust (strict)"(error in=w389, "DisabledEnum"=w388) -> (error out=w370:errorcluster)  [unwired: 1 in, 1 out]
        n142 = property on="RFID" class="Bool (strict)"(error in=w370, "BoolText.Text"="" ("Boolean Text.Text")) -> (error out=w368:errorcluster)  [unwired: 1 in, 1 out]
        n143 = property on="RFID" class="Bool (strict)"(error in=w368, "Colors [4]"=cluster{u32, u32}[] [{0, 0}]) -> (error out=w366:errorcluster)  [unwired: 1 in, 1 out]
      }
      frame "Alert Owner" {
        # "Path to store Image taken."
        # "Build path to send image to \nOwner."
        # "Close Camera."
        # "Take Picture of  intruder \nand save image."
        # "Open Camera."
        # "Send message to owner."
        n144 = call <vilib>:"IMAQdx Open Camera.vi"("error in"=w436, "Session In"=T15 "cam0") -> ("error out"=w447:errorcluster, "Session Out"=w448:T15)  [unwired: 8 in]
        n145 = call "Capture Intruder.vi"("File Path"=path "C:/Users/jmart/OneDrive/Documents/College assignments/UCSD/ECE 144/Intruder.png", "error in"=w447, "Session In"=w448) -> ("error out"=w446:errorcluster, "Image"=w442:T3, "Session Out"=w443:T15, "File Path"=w439:path)  [unwired: 5 in]
        n146 = call <vilib>:"IMAQdx Close Camera.vi"("error in"=w446, "Session In"=w443) -> ("error out"=w440:errorcluster)  [unwired: 9 in]
        n147 = Build Array(w439) -> (w438:path[])
        n148 = call "SMTP.vi"("Carrier"=T16."T-Mobile", "Outgoing Mail Server (SMTP)"="smtp.gmail.com", "Email"="ece144.smtp@gmail.com", "Password"="LabVIEW_Texting", "Phone Number"="5626595947", "Subject"="House Alarm Triggered.", "Body"="Jaime! Someone has\nset the alarm too many\ntimes. Police was\ncontacted.", "attachments"=w438) -> ("error out"=w445:errorcluster)  [unwired: 11 in]
        n149 = Merge Errors(w445, w440) -> (w444:errorcluster)
      }
      frame "Turn Off LED" {
        w468 = FALSE ("Granted")
        # "Turn off RFID indicator & \nturn off text"
        # "Turn off LEDs from RGB"
        # "Turn off all LEDs on Front panel and RGB from hardware."
        n150 = Unbundle By Name(w478) -> ("RGB"=w477:u8[])
        n151 = call-poly <vilib>:"Digital Write.vi"("Error In"=w474, "Values"=bool[] [FALSE, FALSE, FALSE], "DO Channels"=w477, "LINX Resource"=w476) -> ("Error Out"=w469:errorcluster, "LINX Resource"=w475:T8)  [unwired: 6 in]
        n152 = property on="Granted" class="Bool (strict)"(error in=w469, "Value"=w468) -> (error out=w467:errorcluster)  [unwired: 1 in, 1 out]
        n153 = property on="Denied" class="Bool (strict)"(error in=w467, "Value"=w468) -> (error out=w465:errorcluster)  [unwired: 1 in, 1 out]
        n154 = property on="RFID" class="Bool (strict)"(error in=w465, "Colors [4]"=cluster{u32, u32}[] [{197379, 0}]) -> (error out=w463:errorcluster)  [unwired: 1 in, 1 out]
        n155 = property on="RFID" class="Bool (strict)"(error in=w463, "BoolText.Text"="" ("Boolean Text.Text")) -> (error out=w462:errorcluster)  [unwired: 1 in, 1 out]
      }
      frame "Stop" {
        w481 = Enum_Control."Stop"  # Initital State
        # "Reset Counter."
        # "Reset passcode"
        # "Stop the program"
      }
    }
    "Passcode Entered" <- w42
    n156 = call "IMAQ Dispose"("All Images? (No)"=TRUE, "error in (no error)"=w27) -> ("error out"=w26:errorcluster)  [unwired: 4 in]
    n157 = local write "Door Animation"(0) -> ()
    n158 = local write "Image"(w29) -> ()
    n159 = call "Liquid Crystal Display.vi"("LINX Resource In"=w36, "Clear LCD?"=u16 4 ("Custom Command Number"), "Error In"=w26) -> ("LINX Resource Out"=w37:T8, "Error Out"=w39:errorcluster)  [unwired: 12 in, 3 out]
  }
  n160 = call-poly <vilib>:"Servo Close.vi"("Error In"=w5, "Servo Channel"=u8 3, "LINX Resource"=w2) -> ("Error Out"=w6:errorcluster, "LINX Resource"=w1:T8)  [unwired: 7 in]
  n161 = Merge Errors(w6, w4) -> (w18:errorcluster)
  n162 = call <vilib>:"Close.vi"("Error In"=w18, "LINX Resource"=w1) -> ("Error Out"=w17:errorcluster)  [unwired: 9 in]
  n163 = call <vilib>:"Simple Error Handler.vi"("error in (no error)"=w17) -> ()  [unwired: 4 in, 5 out]
